vi "Shared Downcast Object.vi"(8 "error in (no error)":errorcluster, 9 "Data Type":u8(ring)=2 items=["DTYPE_BU"=2, "DTYPE_WU"=3, "DTYPE_LU"=4, "DTYPE_QU"=5, "DTYPE_OU"=25, "DTYPE_B"=6, "DTYPE_W"=7, "DTYPE_L"=8, "DTYPE_Q"=9, "DTYPE_O"=26, "DTYPE_FLOAT"=52, "DTYPE_DOUBLE"=53, "DTYPE_T"=14, "DTYPE_IDENT"=191, "DTYPE_NID"=192, "DTYPE_PATH"=193, "DTYPE_PARAM"=194, "DTYPE_SIGNAL"=195, "DTYPE_DIMENSION"=196, "DTYPE_WINDOW"=197, "DTYPE_SLOPE"=198, "DTYPE_FUNCTION"=199, "DTYPE_CONGLOM"=200, "DTYPE_RANGE"=201, "DTYPE_ACTION"=202, "DTYPE_DISPATCH"=203, "DTYPE_PROGRAM"=204, "DTYPE_ROUTINE"=205, "DTYPE_PROCEDURE"=206, "DTYPE_METHOD"=207, "DTYPE_DEPENDENCY"=208, "DTYPE_CONDITION"=209, "DTYPE_EVENT"=210, "DTYPE_WITH_UNITS"=211, "DTYPE_CALL"=212, "DTYPE_WITH_ERROR"=213, "DTYPE_LIST"=214, "DTYPE_TUPLE"=215, "DTYPE_DICTIONARY"=216, "DTYPE_POINTER"=51, "DTYPE_DSC"=24], 10 "Class Type":u8(ring)=2 items=["CLASS_S"=1, "CLASS_D"=2, "CLASS_A"=4, "CLASS_R"=194, "CLASS_APD"=196], 11 "Data in":refnum<class "Data.lvclass">) -> (0 "error out":errorcluster, 3 "Data out":refnum<class "Data.lvclass">)   [LabVIEW 2012, in "MDSplus.lvlib" / "Data.lvclass"]
uses:
  <vilib>/MDSplus/Classes/Data_Class/Data.lvclass
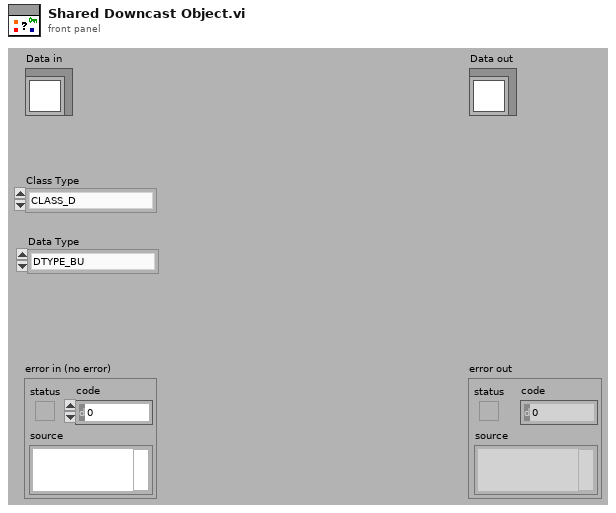
[diagram p1: front panel]
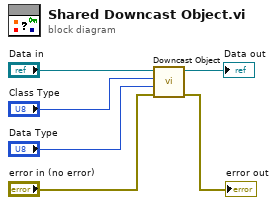
[diagram p0: block diagram]
diagram:
  n1 = call <vilib>:"Downcast Object.vi"("error in (no error)"="error in (no error)", "Data Type"="Data Type", "Class Type"="Class Type", "Data in"="Data in") -> ("error out"=→"error out":errorcluster, "Data out"=→"Data out":refnum<class "Data.lvclass">)  [unwired: 6 in]
